vi "PH_Calorimeter_USB.constructor.vi"(0 "name":string, 2 "data in":string, 5 "error in(no error)":errorcluster) -> (14 "i ref out":refnum<vi>, 16 "data out":string, 19 "error out":errorcluster)   [LabVIEW 2014, in "PH_Calorimeter_USB.lvlib"]
doc: "This class is forseen to get the data and to calculate the energy of the calorimeter which are taken by the use of a NI USB-6009 I/O device.\n\nThis class is part of the PHELIX user layer.\n\nauthor: Stefan Götte, GSI\n\nLicense Agreement for this software:\n\nCopyright (C)\nGesellschaft für Schwerionenforschung, GSI\nPlanckstr. 1\n64291 Darmstadt\nGermany\n\nContact: D.Beck@gsi.de \n\nThis program is free software; you can redistribute it and/or modify it under the terms of the \nGNU General Public License as published by the Free Software Foundation; either version 2 of \nthe license, or (at your option) any later version.\n\nThis program is distributed in the hope that it will be useful, but WITHOUT ANY WARRANTY; \nwithout even the implied warranty of MERCHANTABILITY or FITNESS FOR A PARTICULAR PURPOSE. See the GNU General License for more details (http://www.gnu.org).\n\nGesellschaft für Schwerionenforschung, GSI\nPlanckstr. 1, 64291 Darmstadt, Germany\nFor all questions and ideas contact: M.Richter@gsi.de, H.Brand@gsi.de or D.Beck@gsi.de.\nLast update: 16-JUN-2004"
uses:
  PH_Calorimeter_USB.lvlib
  PH_Basics/PH_PSDBWriter/PH_PSDBWriter.lvlib
  PH_Basics/PH_Class/PH_Class.lvlib
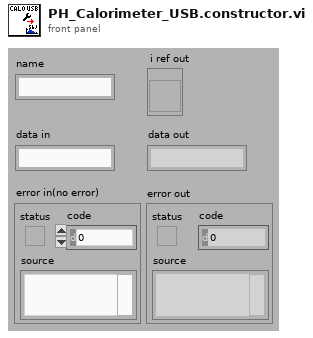
[diagram p1: front panel]
types:
  T1 = enum16{"SetAttribute", "GetAttribute", "CreateAttribute", "DestroyAttribute", "DestroyAllAtributes"}
  T2 = typedef "PH_Calorimeter_USB.lvlib/PH_Calorimeter_USB.i attribute.ctl" = cluster{"GUI Refs":cluster{"Delete":refnum<vi>, "Start":refnum<vi>, "Energy":refnum<vi>, "Calorimeter":refnum<vi>, "Trigger":refnum<vi>, "Calo Calibration":refnum<vi>, "Time Base":refnum<vi>, "Device":refnum<vi>, "Graph Raw Data":refnum<vi>, "Graph Result":refnum<vi>}, "DAQ Instance":string, "Data":dbl[][], "Controller Instance":string, "Energy [J]":dbl, "Calorimeter":T3, "Trigger":T4, "Time Base":T5, "Calo Calibration":T6, "Serial Number":string}
  T3 = typedef "PH_Calorimeter_USB.lvlib/PH_Calorimeter_USB.Calorimeter Settings.ctl" = cluster{"Channel":tag, "Min Value [V]":dbl, "Max Value  [V]":dbl}
  T4 = typedef "PH_Calorimeter_USB.lvlib/PH_Calorimeter_USB.Trigger Settings.ctl" = cluster{"Channel":tag, "Min Value [V]":dbl, "Max Value  [V]":dbl, "Level [V]":dbl, "Wait Time [s]":dbl, "Length [Samples]":i32}
  T5 = typedef "PH_Calorimeter_USB.lvlib/PH_Calorimeter_USB.Time Base Settings.ctl" = cluster{"Samples per Channel":i32, "Rate [Hz]":i32}
  T6 = typedef "PH_Calorimeter_USB.lvlib/PH_Calorimeter_USB.Calorimeter Calibration Settings.ctl" = cluster{"T 1/e [s]":dbl, "Sensitivity  [Vs/J]":dbl}
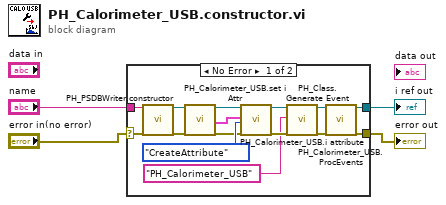
[diagram p0: block diagram]
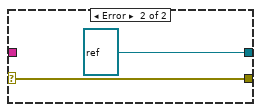
[diagram p2: hidden frame]
diagram:
  n1 = case shown="No Error" "error in(no error)" {
    selector: "error in(no error)" -> [w5 w21]
    tunnel: "name" -> [w19 _]
    tunnel: [w12 w21] -> w3
    tunnel: [w15 refnum<vi> refnum ("i ref out")] -> w2
    frame No Error {
      n2 = call "PH_PSDBWriter.constructor.vi"("name"=w19, "error in"=w5) -> ("i ref out"=w10:refnum<vi>, "error out"=w8:errorcluster)  [unwired: 15 in, 1 out]
      n3 = call "PH_Calorimeter_USB.set i Attr.vi"("i ref in"=w10, "error in (no error)"=w8) -> ("i ref out"=w9:refnum<vi>, "i Attributes"=w6:T2, "error out"=w7:errorcluster)  [unwired: 15 in]
      n4 = call "PH_Calorimeter_USB.i attribute.vi"("VI Refnum"=w9, "CLASS.i attribute"=w6, "Action"=T1."CreateAttribute", "error in (no error)"=w7) -> ("VI Refnum out"=w17:refnum<vi>, "error out"=w14:errorcluster)  [unwired: 13 in, 1 out]
      n5 = call "PH_Class.Generate Event.vi"("i ref in"=w17, "Class"="PH_Calorimeter_USB", "error in (no error)"=w14) -> ("i ref out"=w16:refnum<vi>, "error out"=w13:errorcluster)  [unwired: 15 in]
      n6 = call "PH_Calorimeter_USB.ProcEvents.vi"("i ref in"=w16, "error in"=w13) -> ("i ref out"=w15:refnum<vi>, "error out"=w12:errorcluster)  [unwired: 16 in]
    }
    frame Error {
    }
  }
  "i ref out" <- w2
  "error out" <- w3
